vi "WritemmWavePositions.vi"(8 "error in (no error)":errorcluster, 9 "mmWave names, positions":T1, 11 "UI MotionStatus in":refnum<class "UI MotionStatus.lvclass">) -> (0 "error out":errorcluster, 3 "UI MotionStatus out":refnum<class "UI MotionStatus.lvclass">)   [LabVIEW 2019, in "UI MotionStatus.lvclass"]
uses:
  UI MotionStatus.lvclass
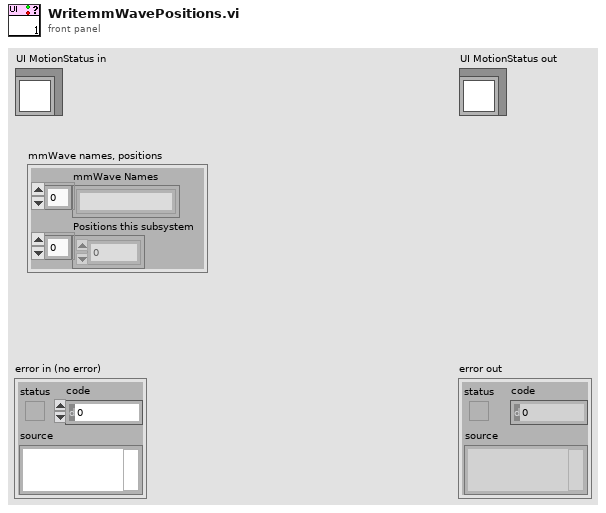
[diagram p1: front panel]
types:
  T1 = cluster{"mmWave Names":string[], "Positions this subsystem":dbl[]}
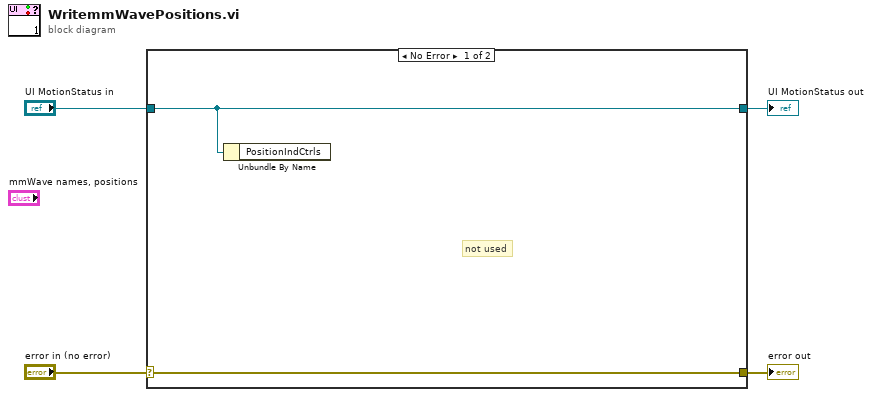
[diagram p0: block diagram]
diagram:
  n1 = case shown="No Error" "error in (no error)" {
    selector: "error in (no error)" -> [w6 w8]
    tunnel: [w6 w8] -> w3
    tunnel: [w5 w7] -> w1
    tunnel: "UI MotionStatus in" -> [w5 w7]
    frame No Error {
      # "not used"
      n2 = Unbundle By Name(w5) -> ()  [unwired: 1 out]
    }
    frame Error {
    }
  }
  "error out" <- w3
  "UI MotionStatus out" <- w1
